vi "Select Project Item Creator.vi"(8 "Error In":errorcluster, 10 "ProjectItem Refnum":refnum<vi>, 11 "Project Items In":T1[](array[typedef])) -> (0 "Error Out":errorcluster, 3 "Project Items Out":T1[](array[typedef]))   [LabVIEW 2014, in "i3-docs.lvlib"]
uses:
  i3-docs.lvlib
  Controls/project_item.ctl
  Controls/image_information.ctl
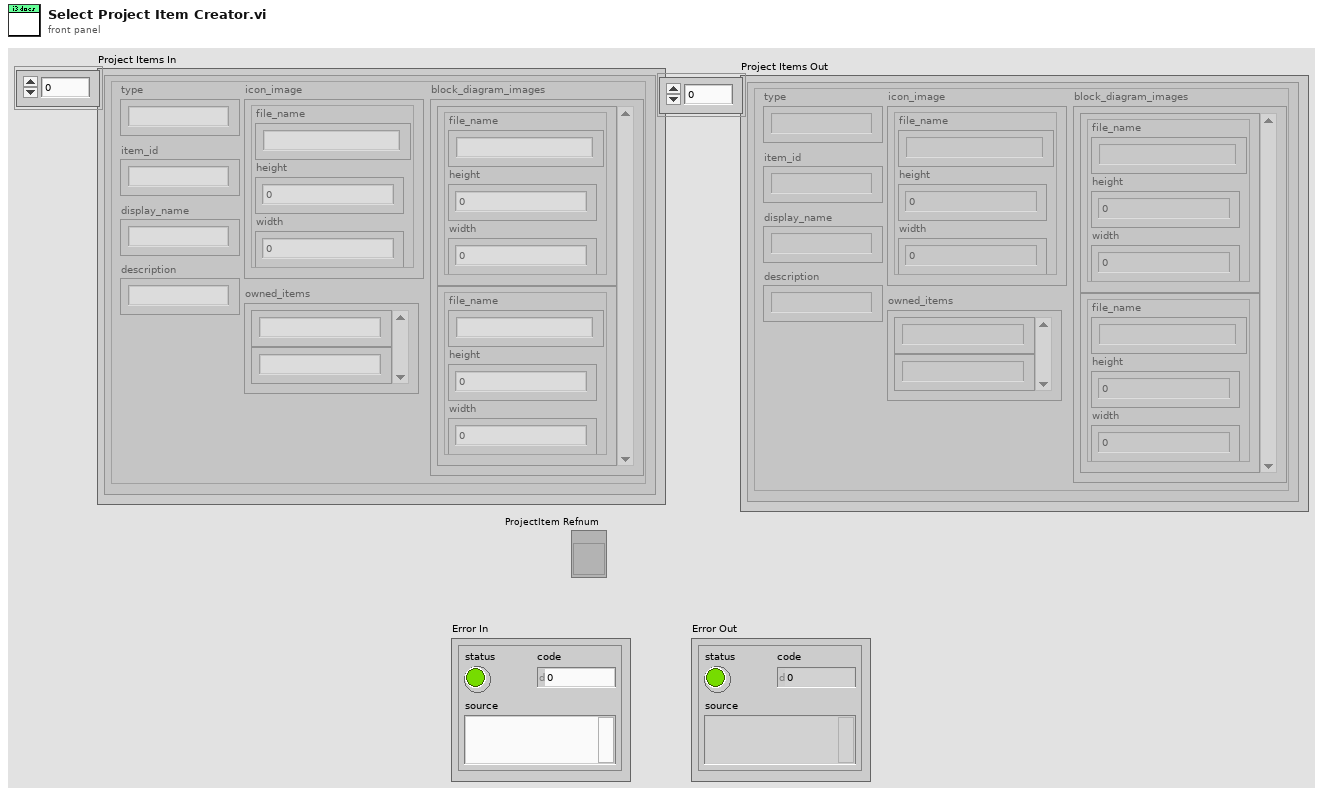
[diagram p1: front panel]
types:
  T1 = typedef "i3-docs.lvlib/project_item.ctl" = cluster{"type":string, "owned_items":string[], "item_id":string, "display_name":string, "description":string, "block_diagram_images":T2[], "icon_image":T2}
  T2 = typedef "i3-docs.lvlib/image_information.ctl" = cluster{"file_name":string, "height":i32, "width":i32}
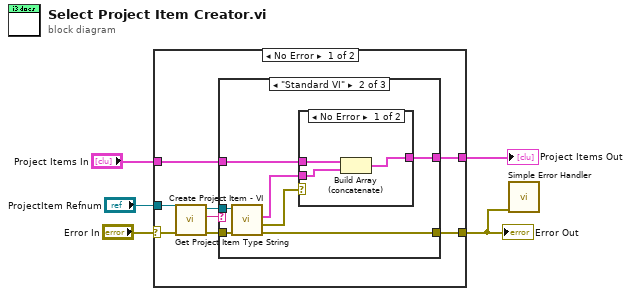
[diagram p0: block diagram]
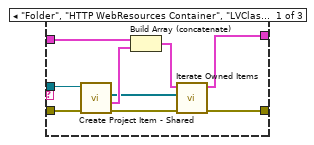
[diagram p2: hidden frame]
diagram:
  n1 = case shown="No Error" "Error In" {
    selector: "Error In" -> [w10 w37]
    tunnel: "ProjectItem Refnum" -> [w6 _]
    tunnel: "Project Items In" -> [w13 w36]
    tunnel: [w11 w36] -> w2
    tunnel: [w12 w37] -> w1
    frame No Error {
      n2 = call "Get Project Item Type String.vi"("Error In"=w10, "ProjectItem Refnum"=w6) -> ("Error Out"=w9:errorcluster, "Type String"=w7:string, "ProjectItem Refnum Out"=w8:refnum<vi>)  [unwired: 7 in]
      n3 = case shown="\"Standard VI\"" w7 {
        tunnel: [w22 w23 w34] -> w12
        tunnel: w13 -> [w19 w28 w35]
        tunnel: [w17 w29 w35] -> w11
        tunnel: w9 -> [w21 w25 w34]
        tunnel: w8 -> [w20 w27 _]
        frame "Folder", "HTTP WebResources Container", "LVClass", "Library", "Startup VIs Container", "Web Service" {
          n4 = call "Create Project Item - Shared.vi"("Error In"=w21, "ProjectItem Refnum"=w20) -> ("Error Out"=w14:errorcluster, "project_item"=w16:T1, "Owned Items[]"=w15:refnum<vi>[])  [unwired: 6 in, 1 out]
          n5 = Build Array (concatenate)(w19, w16) -> (w18:T1[])
          n6 = call "Iterate Owned Items.vi"("Error In"=w14, "Owned Items[]"=w15, "Project Items In"=w18) -> ("Error Out"=w22:errorcluster, "Project Items Out"=w17:T1[])  [unwired: 7 in]
        }
        frame "Standard VI" {
          n7 = call "Create Project Item - VI.vi"("Error In"=w25, "ProjectItem Refnum"=w27) -> ("Error Passthrough"=w23:errorcluster, "Error During VI Project Item Creation"=w24:errorcluster, "Project Item Out"=w26:T1)  [unwired: 6 in, 1 out]
          n8 = case shown="No Error" w24 {
            tunnel: [w32 w33] -> w29
            tunnel: w28 -> [w31 w33]
            tunnel: w26 -> [w30 _]
            frame No Error {
              n9 = Build Array (concatenate)(w31, w30) -> (w32:T1[])
            }
            frame Error {
            }
          }
        }
        frame Default {
        }
      }
    }
    frame Error {
    }
  }
  "Project Items Out" <- w2
  "Error Out" <- w1
  n10 = call <vilib>:"Simple Error Handler.vi"("error in (no error)"=w1) -> ()  [unwired: 4 in, 5 out]
